vi "refresh program list.vi"(8 "error in (no error)":errorcluster, 10 "reference":refnum<vi>, 11 "Programs in":refnum<class "Programs.lvclass">) -> (0 "error out":errorcluster, 2 "Program List":string[](array[string]), 3 "Programs out":refnum<class "Programs.lvclass">)   [LabVIEW 2025, in "Programs.lvclass"]
uses:
  Programs.lvclass
  Programs.lvclass/Programs.ctl
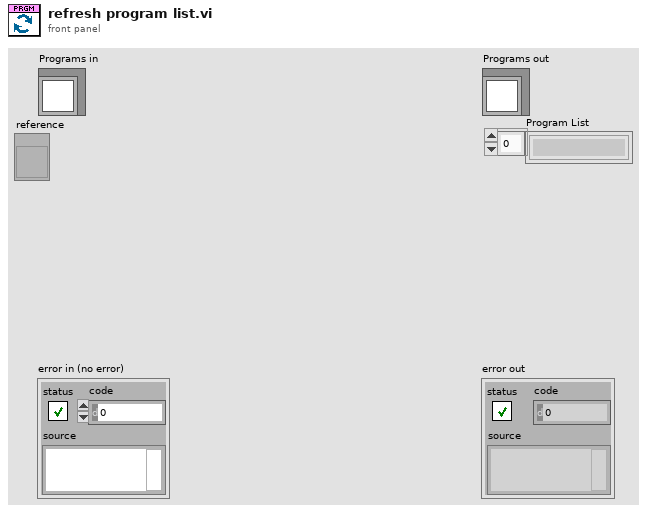
[diagram p1: front panel]
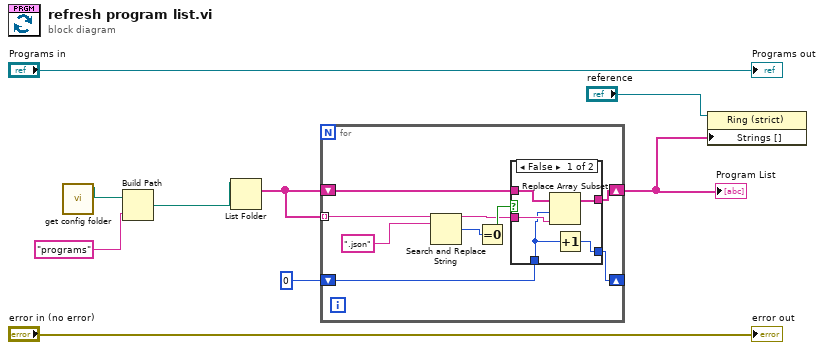
[diagram p0: block diagram]
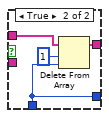
[diagram p2: hidden frame]
diagram:
  n1 = call "get config folder.vi"() -> ("Config folder path"=w3:path)  [unwired: 11 in]
  n2 = Build Path(base path=w3, name or relative path="programs") -> (appended path=w1:path)
  n3 = List Folder(path=w1) -> (filenames=w7:string[])  [unwired: 3 in, 3 out]
  n4 = for {
    shift-right: [w13] -> w5
    shift-left: w7 -> [w15]
    tunnel: w7 -> [w18] mode=indexing
    shift-right: [w10] -> _
    shift-left: 0 ("index") -> [w11]
    n5 = Search and Replace String(input string=w18, search string=".json") -> (result string=w12:string, number of replacements=w16:i32)  [unwired: 6 in, 2 out]
    n6 = Equal To 0?(x=w16) -> (x = 0?=w14:bool)
    n7 = case shown="False" w14 {
      tunnel: w15 -> [w23 w27]
      tunnel: [w21 w25] -> w13
      tunnel: w12 -> [w22 _]
      tunnel: w11 -> [w19 w24]
      tunnel: [w20 w24] -> w10
      frame False {
        n8 = Replace Array Subset(array=w23, new element=w22, index=w19) -> (w21:string[])
        n9 = Increment(x=w19) -> (x+1=w20:i32)
      }
      frame True {
        n10 = Delete From Array(array=w27, length=1, index=w24) -> (array with subset deleted=w25:string[])  [unwired: 1 out]
      }
    }
  }
  "Program List" <- w5
  n11 = property on="Property Node" class="Ring (strict)"(reference="reference", "Strings []"=w5) -> ()  [unwired: 1 in, 2 out]
  "error out" <- "error in (no error)"
  "Programs out" <- "Programs in"
